vi "Go To Rotator Position.vi"(8 "error in (no error)":errorcluster, 10 "Position (deg)":dbl=90.0) -> (0 "error out":errorcluster)   [LabVIEW 2016]
uses:
  PPMS Global.vi
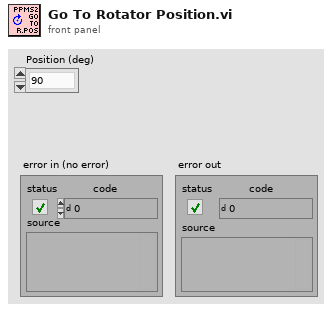
[diagram p1: front panel]
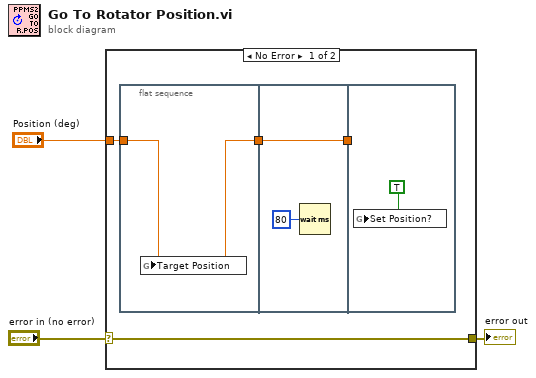
[diagram p0: block diagram]
diagram:
  n1 = case shown="No Error" "error in (no error)" {
    selector: "error in (no error)" -> [w7 w12]
    tunnel: [w7 w12] -> w2
    tunnel: "Position (deg)" -> [w6 _]
    frame No Error {
      n2 = flat-sequence {
        tunnel: w6 -> [w8]
        tunnel: [w8] -> w4
        tunnel: [w9] -> w5
        tunnel: w4 -> [w9]
        tunnel: w5 -> [_]
        frame #0 {
          n3 = global write "PPMS Global.vi" "Target Position"(w8) -> ()
        }
        frame #1 {
          n4 = Wait (ms)(milliseconds to wait=u32 80) -> ()  [unwired: 1 out]
        }
        frame #2 {
          n5 = global write "PPMS Global.vi" "Set Position?"(TRUE ("Set Field?")) -> ()
        }
      }
    }
    frame Error {
    }
  }
  "error out" <- w2
